vi "Simple Add.vi"(9 "Numeric 3":dbl, 10 "Numeric 2":dbl, 11 "Numeric 1":dbl) -> (3 "x+y":dbl)   [LabVIEW 2019]
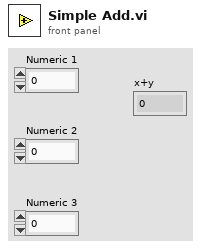
[diagram p1: front panel]
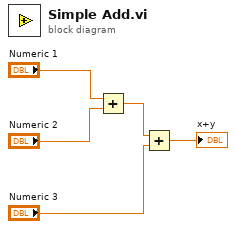
[diagram p0: block diagram]
diagram:
  n1 = Add(x="Numeric 1", y="Numeric 2") -> (x+y=w3:dbl)
  n2 = Add(x=w3, y="Numeric 3") -> (x+y=→"x+y":dbl)
